vi "New.vi"(10 "Min":dbl, 11 "Max":dbl) -> (3 "ConfigA.lvclass":refnum<class "ConfigA.lvclass">)   [LabVIEW 2019, in "ConfigA.lvclass"]
uses:
  ConfigA.lvclass
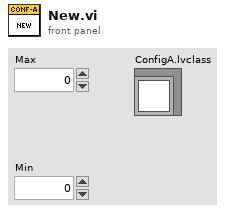
[diagram p1: front panel]
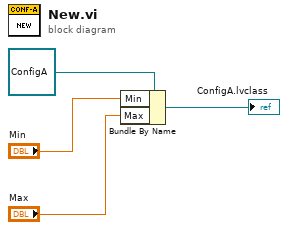
[diagram p0: block diagram]
diagram:
  n1 = Bundle By Name(cluster=refnum<class "ConfigA.lvclass"> refnum ("ConfigA.lvclass"), "Min"="Min", "Max"="Max") -> (→"ConfigA.lvclass":refnum<class "ConfigA.lvclass">)
